vi "WaveRunner.vi"(5 "error out":errorcluster, 7 "Sequence Number":i32, 9 "actual  record length":i32, 10 "Channel name":string, 11 "instrument handle out":refnum<k15>) -> (0 "error in (no error)":errorcluster, 1 "initial x":dbl format="%.2f", 2 "element value":dbl format="%.2f", 3 "instrument handle":refnum<k15>, 4 "waveform array":dbl[](array[numeric]) format="%.2f", 8 "Actual Pts":i32)   [LabVIEW 2022 SP3]
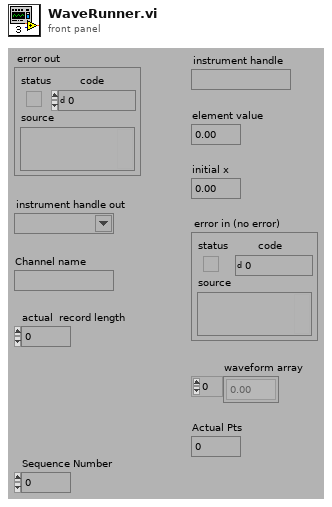
[diagram p1: front panel]
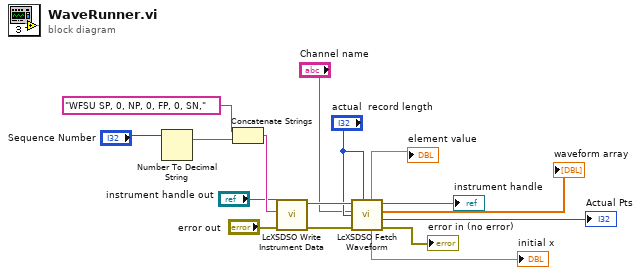
[diagram p0: block diagram]
diagram:
  n1 = Number To Decimal String(number="Sequence Number") -> (decimal integer string=w15:string)  [unwired: 1 in]
  n2 = Concatenate Strings("WFSU SP, 0, NP, 0, FP, 0, SN,", w15) -> (w16:string)
  n3 = call "LcXSDSO Write Instrument Data.vi"("error in (no error)"="error out", "write buffer"=w16, "instrument handle"="instrument handle out") -> ("error out"=w12:errorcluster, "instrument handle out"=w13:refnum<k15>)  [unwired: 7 in]
  n4 = call "LcXSDSO Fetch Waveform.vi"("size of waveform array"="actual  record length", "error in (no error)"=w12, "waveform size"="actual  record length", "channel name"="Channel name", "instrument handle"=w13) -> ("error out"=→"error in (no error)":errorcluster, "actual points"=→"Actual Pts":i32, "waveform array"=→"waveform array":dbl[], "instrument handle out"=→"instrument handle":refnum<k15>, "initial x"=→"initial x":dbl, "x increment"=→"element value":dbl)  [unwired: 1 in]
